vi "06.2 Handle Specific Errors Immediately.vi"() -> ()   [LabVIEW 2019]
uses:
  Support Files/02.4 DAQmx Configuration Cluster.ctl
  Support Files/03.2 States.ctl
  Support Files/03.2 State Machine Data.ctl
  <vilib>/DAQmx/read.llb/DAQmx Read (Analog 2D DBL NChan NSamp).vi
  <vilib>/DAQmx/write.llb/DAQmx Write (Analog DBL 1Chan 1Samp).vi
  <vilib>/DAQmx/create/channels.llb/DAQmx Create Channel (AI-Voltage-Basic).vi
  <vilib>/DAQmx/configure/timing.llb/DAQmx Timing (Sample Clock).vi
  <vilib>/DAQmx/miscellaneous.llb/DAQmx Fill In Error Info.vi
  <vilib>/Utility/file.llb/Write Delimited Spreadsheet (string).vi
  <vilib>/Utility/file.llb/Write Delimited Spreadsheet (DBL).vi
  <vilib>/DAQmx/create/channels.llb/DAQmx Create Channel (AO-Voltage-Basic).vi
panel:
  in  "DAQmx Configuration Cluster":T1={"Desired Sample Rate (Hz)"=-1.0, "sample mode"=10178, "Minimum value"=-1.0, "Maximum value"=-1.0, "Physical Channel"="", "units"=10143, "thermocouple type"=10072, "Samples per Channel"=0} {"thermocouple type" items=["J"=10072, "K"=10073, "N"=10077, "R"=10082, "S"=10085, "T"=10086, "B"=10047, "E"=10055]; "units" items=["Deg C"=10143, "Deg F"=10144, "Kelvins"=10325, "Deg R"=10145, "From Custom Scale"=10065]; "sample mode" items=["Finite Samples"=10178, "Continuous Samples"=10123, "Hardware Timed Single Point"=12522]}
  in  "Threshold (RMS)":dbl
  in  "Generate Stimulus":bool
  in  "Stop":bool
  in  "Clear":bool
  in  "Acquire":bool
  out "Graph":dbl[][](graph)
  out "Thershold Exceeded?":bool
  out "RMS Result per Channel":dbl[](array[numeric])
  # "ANALYSIS"
  # "EVENTS"
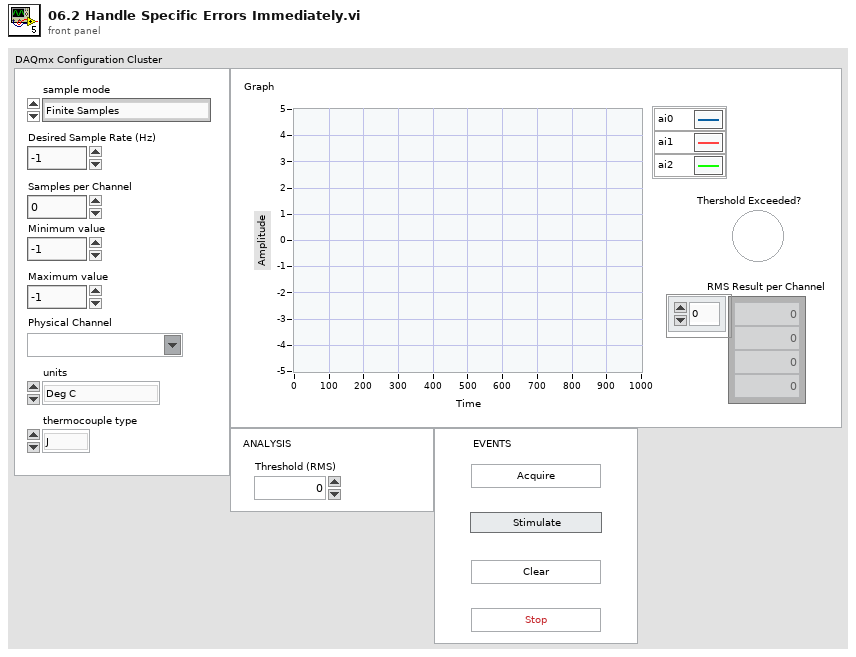
[diagram p1: front panel]
types:
  T1 = typedef "02.4 DAQmx Configuration Cluster.ctl" = cluster{"Desired Sample Rate (Hz)":dbl, "sample mode":i32, "Minimum value":dbl, "Maximum value":dbl, "Physical Channel":tag, "units":i32, "thermocouple type":i32, "Samples per Channel":i32}
  T2 = typedef "03.2 State Machine Data.ctl" = cluster{"Acquisition Data":dbl[][], "Stimulus?":bool}
  T3 = typedef "03.2 States.ctl" = enum16{"Initialize", "Update UI", "Update Stimulus", "Wait for event", "Acquire", "Analyze", "Log", "Clear", "Shutdown"}
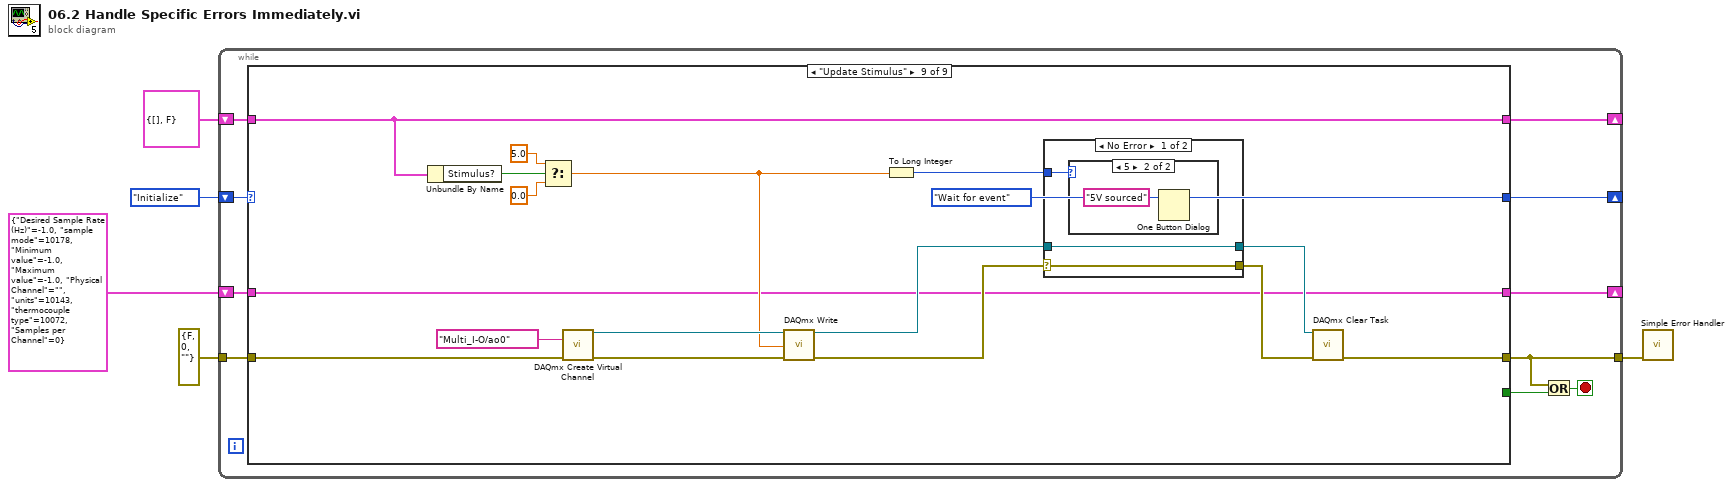
[diagram p0: block diagram]
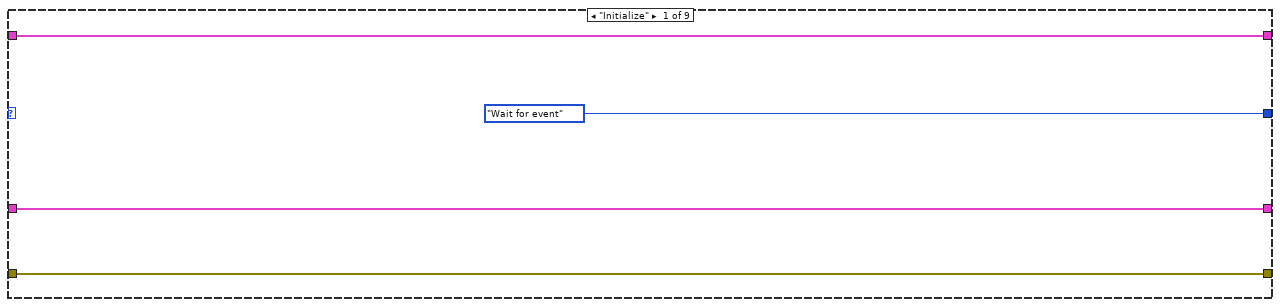
[diagram p2: hidden frame]
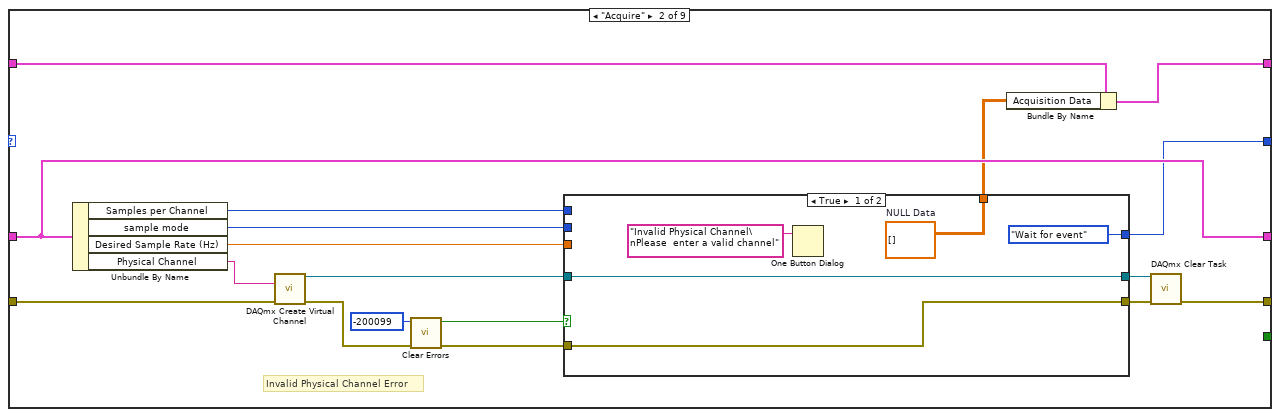
[diagram p3: hidden frame]
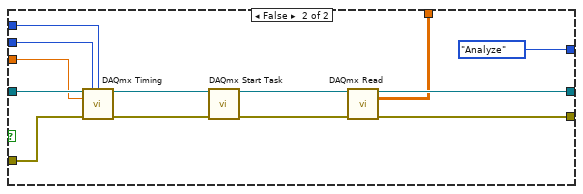
[diagram p4: hidden frame]
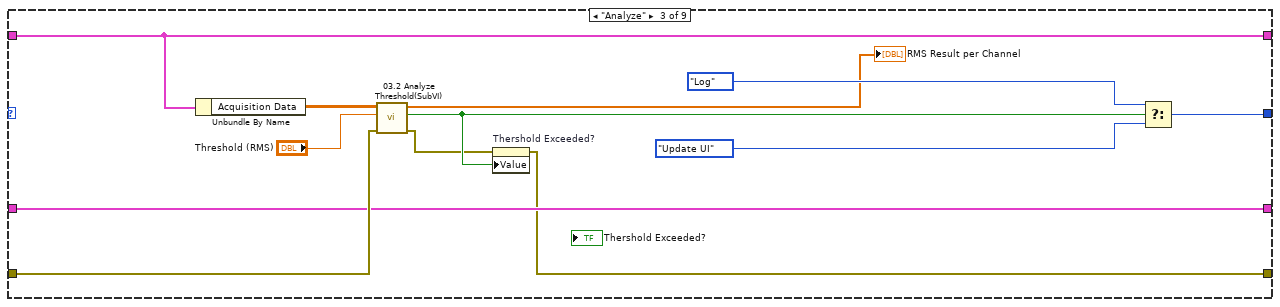
[diagram p5: hidden frame]
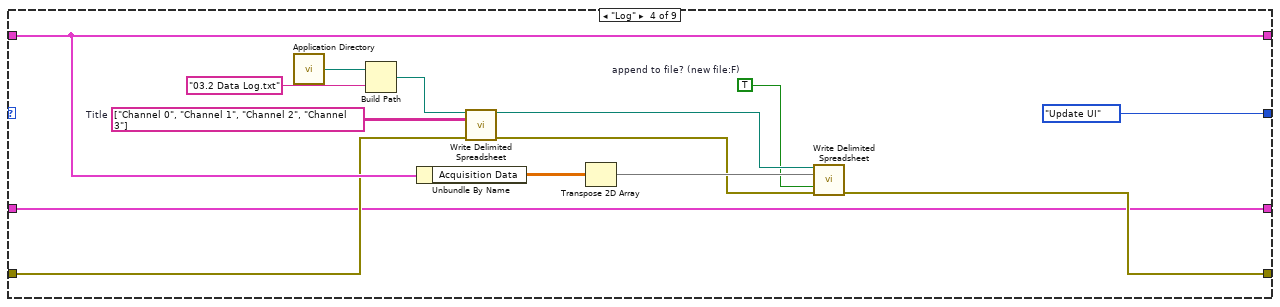
[diagram p6: hidden frame]
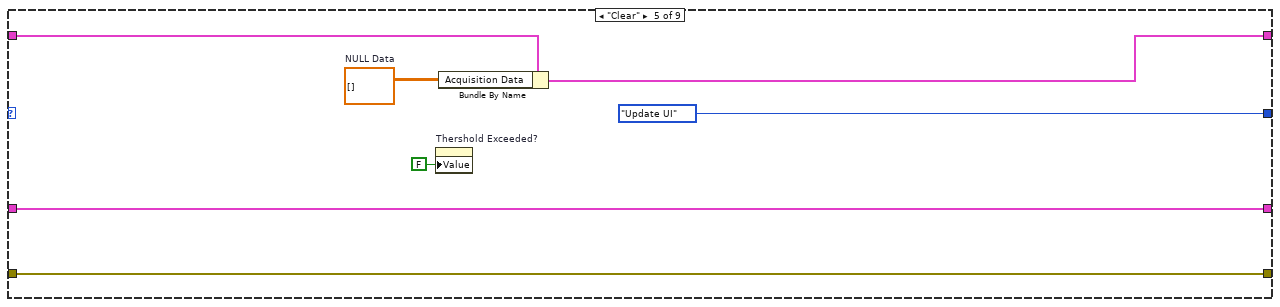
[diagram p7: hidden frame]
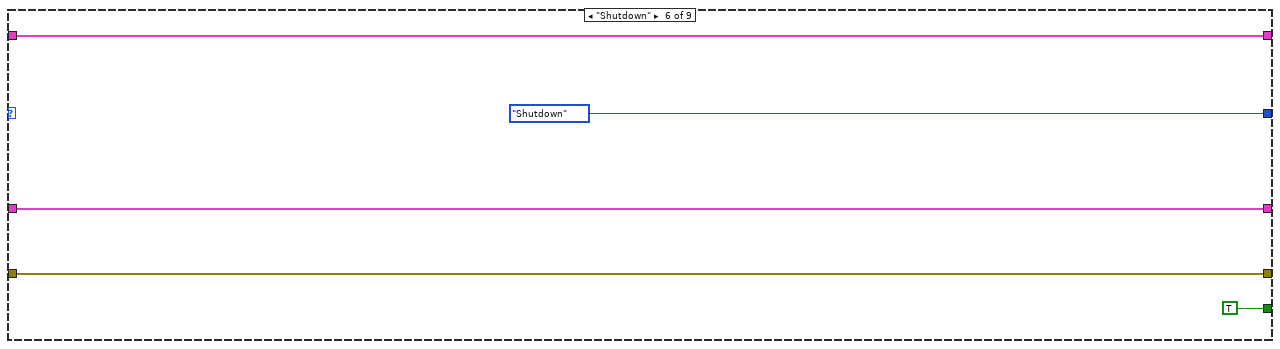
[diagram p8: hidden frame]
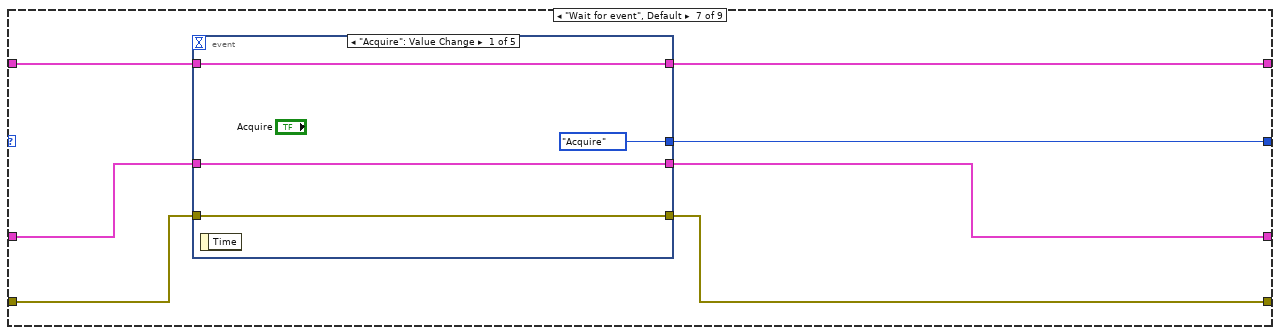
[diagram p9: hidden frame]
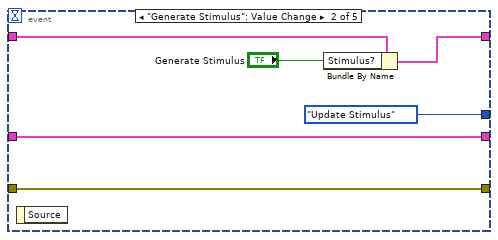
[diagram p10: hidden frame]
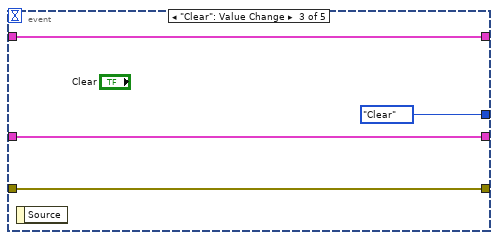
[diagram p11: hidden frame]
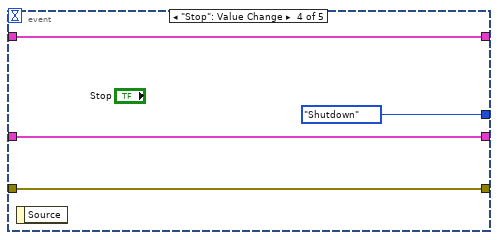
[diagram p12: hidden frame]
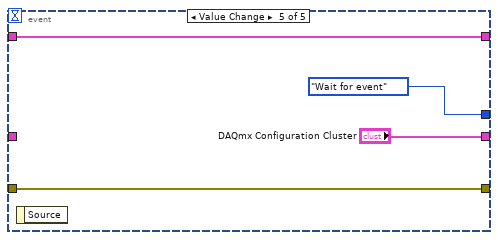
[diagram p13: hidden frame]
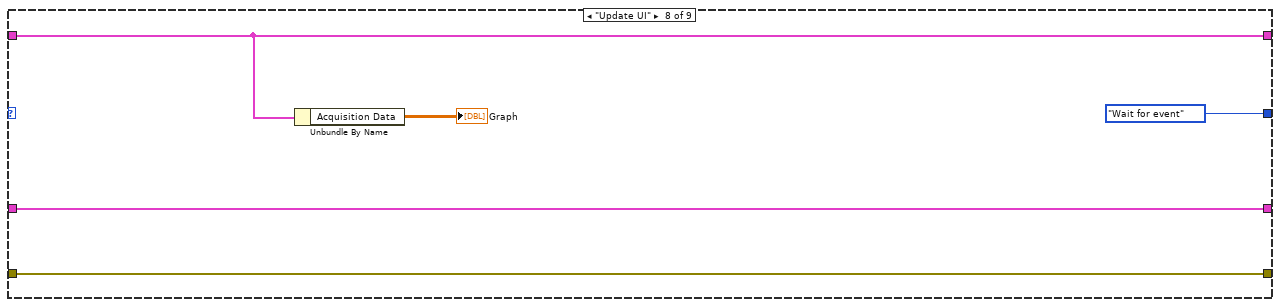
[diagram p14: hidden frame]
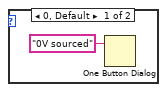
[diagram p15: hidden frame]
diagram:
  n1 = while {
    shift-right: [w14] -> _
    shift-left: 03.2_States."Initialize" ("State") -> [w15]
    tunnel: errorcluster {"status"=FALSE, "code"=0, "source"=""} ("error constant") -> [w13]
    tunnel: [w11] -> w3
    shift-right: [w10] -> _
    shift-left: T2 {"Acquisition Data"=[], "Stimulus?"=FALSE} -> [w9]
    shift-right: [w6] -> _
    shift-left: T1 {"Desired Sample Rate (Hz)"=-1.0, "sample mode"=10178, "Minimum value"=-1.0, "Maximum value"=-1.0, "Physical Channel"="", "units"=10143, "thermocouple type"=10072, "Samples per Channel"=0} ("DAQmx Configuration Cluster") -> [w7]
    stop <- w12 stop-if-true
    n2 = case shown="\"Update Stimulus\"" w15 {
      tunnel: [03.2_States."Wait for event" ("State") w20 w66 03.2_States."Update UI" ("State") 03.2_States."Update UI" ("State") 03.2_States."Shutdown" ("State") w100 03.2_States."Wait for event" ("State") 03.2_States."Wait for event" ("State")] -> w14
      tunnel: [w18 w27 w56 w79 w84 w91 w99 w125 w133] -> w11
      tunnel: w13 -> [w18 w32 w63 w69 w84 w91 w98 w125 w144]
      tunnel: [w19 w21 w62 w77 w87 w92 w97 w127 w130] -> w10
      tunnel: w9 -> [w19 w23 w62 w77 w88 w92 w96 w127 w130]
      tunnel: [_ _ _ _ _ TRUE _ _ _] -> w8
      tunnel: w7 -> [w16 w24 w58 w68 w83 w89 w95 w123 w129]
      tunnel: [w16 w24 w58 w68 w83 w89 w94 w123 w129] -> w6
      frame "Initialize" {
      }
      frame "Acquire" {
        # "Invalid Physical Channel Error"
        n3 = Unbundle By Name(w24) -> ("Samples per Channel"=w34:i32, "sample mode"=w35:i32, "Desired Sample Rate (Hz)"=w36:dbl, "Physical Channel"=w33:tag)
        n4 = call-poly <vilib>:"DAQmx Create Virtual Channel.vi"("physical channels"=w33, "error in"=w32) -> ("task out"=w37:refnum<k21>, "error out"=w31:errorcluster)  [unwired: 12 in]
        n5 = call <vilib>:"Clear Errors.vi"("error in (no error)"=w31, "specific error code to clear (0: all)"=-200099) -> ("error out"=w29:errorcluster, "specific error cleared?"=w28:bool)  [unwired: 4 in]
        n6 = case shown="True" w28 {
          tunnel: w29 -> [w41 w55]
          tunnel: w37 -> [w42 w54]
          tunnel: w36 -> [_ w49]
          tunnel: w35 -> [_ w48]
          tunnel: w34 -> [_ w47]
          tunnel: [w41 w46] -> w26
          tunnel: [w42 w45] -> w25
          tunnel: [w40 w44] -> w22
          tunnel: [03.2_States."Wait for event" ("State") 03.2_States."Analyze" ("State")] -> w20
          frame True {
            w40 = dbl[][] []  # NULL Data
            n7 = One Button Dialog(message="Invalid Physical Channel\nPlease  enter a valid channel") -> ()  [unwired: 1 in, 1 out]
          }
          frame False {
            n8 = call-poly <vilib>:"DAQmx Timing.vi"("task/channels in"=w54, "sample mode"=w48, "samples per channel"=w47, "rate"=w49, "error in"=w55) -> ("task out"=w50:refnum<k21>, "error out"=w51:errorcluster)  [unwired: 9 in]
            n9 = call <vilib>:"DAQmx Start Task.vi"("task/channels in"=w50, "error in"=w51) -> ("task out"=w52:refnum<k21>, "error out"=w53:errorcluster)  [unwired: 12 in]
            n10 = call-poly <vilib>:"DAQmx Read.vi"("task/channels in"=w52, "error in"=w53) -> ("task out"=w45:refnum<k21>, "data"=w44:dbl[][], "error out"=w46:errorcluster)  [unwired: 11 in]
          }
        }
        n11 = Bundle By Name(cluster=w23, "Acquisition Data"=w22) -> (w21:T2)
        n12 = call <vilib>:"DAQmx Clear Task.vi"("task in"=w25, "error in"=w26) -> ("error out"=w27:errorcluster)  [unwired: 13 in]
      }
      frame "Analyze" {
        n13 = Unbundle By Name(w62) -> ("Acquisition Data"=w67:dbl[][])
        n14 = call "03.2 Analyze Threshold(SubVI).vi"("Error In"=w63, "Threshold (RMS)"="Threshold (RMS)", "Data"=w67) -> ("Error Out"=w57:errorcluster, "Threshold exceeded?"=w59:bool, "RMS Results per Channel"=→"RMS Result per Channel":dbl[])  [unwired: 6 in]
        n15 = property on="Thershold Exceeded?" class="Bool (strict)"(error in=w57, "Value"=w59) -> (error out=w56:errorcluster)  [unwired: 1 in, 1 out]
        n16 = Select(t=03.2_States."Log" ("State"), s=w59, f=03.2_States."Update UI" ("State")) -> (s? t:f=w66:T3)
      }
      frame "Log" {
        w71 = string[][] [["Channel 0", "Channel 1", "Channel 2", "Channel 3"]]  # Title
        w73 = TRUE  # append to file? (new file:F)
        n17 = call <vilib>:"Application Directory.vi"() -> ("Application Directory"=w81:path)
        n18 = Build Path(base path=w81, name or relative path="03.2 Data Log.txt") -> (appended path=w72:path)
        n19 = Unbundle By Name(w77) -> ("Acquisition Data"=w76:dbl[][])
        n20 = call-poly <vilib>:"Write Delimited Spreadsheet.vi"("file path (dialog if empty)"=w72, "2D data"=w71, "error in (no error)"=w69) -> ("new file path (Not A Path if cancelled)"=w74:path, "error out"=w70:errorcluster)  [unwired: 11 in]
        n21 = Transpose 2D Array(2D array=w76) -> (transposed array=w75:dbl[][])
        n22 = call-poly <vilib>:"Write Delimited Spreadsheet.vi"("file path (dialog if empty)"=w74, "2D data"=w75, "append to file? (new file:F)"=w73, "error in (no error)"=w70) -> ("error out"=w79:errorcluster)  [unwired: 10 in, 1 out]
      }
      frame "Clear" {
        w86 = dbl[][] []  # NULL Data
        n23 = property on="Thershold Exceeded?" class="Bool (strict)"("Value"=FALSE ("Thershold Exceeded?")) -> ()  [unwired: 2 in, 2 out]
        n24 = Bundle By Name(cluster=w88, "Acquisition Data"=w86) -> (w87:T2)
      }
      frame "Shutdown" {
      }
      frame "Wait for event", Default {
        n25 = event shown="[0] \"Acquire\": Value Change" {
          selector: _ -> [_ _ _ _ _]
          dyn-events: _ -> [_ _ _ _ _]
          timeout: _ -> [_ _ _ _ _]
          tunnel: [03.2_States."Acquire" ("State") 03.2_States."Update Stimulus" ("State") 03.2_States."Clear" ("State") 03.2_States."Shutdown" ("State") 03.2_States."Wait for event" ("State")] -> w100
          tunnel: [w103 w106 w112 w117 w119] -> w99
          tunnel: w98 -> [w103 w106 w112 w117 w119]
          tunnel: [w102 w108 w114 w116 w121] -> w97
          tunnel: w96 -> [w102 w110 w114 w116 w121]
          tunnel: w95 -> [w101 w105 w111 w115 _]
          tunnel: [w101 w105 w111 w115 "DAQmx Configuration Cluster"] -> w94
          event "Acquire": Value Change {
            n26 = event-data() -> ()  [unwired: 1 in, 1 out]
          }
          event "Generate Stimulus": Value Change {
            n27 = event-data() -> ()  [unwired: 1 in, 1 out]
            n28 = Bundle By Name(cluster=w110, "Stimulus?"="Generate Stimulus") -> (w108:T2)
          }
          event "Clear": Value Change {
            n29 = event-data() -> ()  [unwired: 1 in, 1 out]
          }
          event "Stop": Value Change {
            n30 = event-data() -> ()  [unwired: 1 in, 1 out]
          }
          event Value Change {
            n31 = event-data() -> ()  [unwired: 1 in, 1 out]
          }
        }
      }
      frame "Update UI" {
        n32 = Unbundle By Name(w127) -> ("Acquisition Data"=→"Graph":dbl[][])
      }
      frame "Update Stimulus" {
        n33 = Unbundle By Name(w130) -> ("Stimulus?"=w141:bool)
        n34 = Select(t=5.0, s=w141, f=0.0) -> (s? t:f=w138:dbl)
        n35 = call-poly <vilib>:"DAQmx Create Virtual Channel.vi"("physical channels"=tag "Multi_I-O/ao0", "error in"=w144) -> ("task out"=w142:refnum<k21>, "error out"=w143:errorcluster)  [unwired: 12 in]
        n36 = call-poly <vilib>:"DAQmx Write.vi"("task/channels in"=w142, "data"=w138, "error in"=w143) -> ("task out"=w136:refnum<k21>, "error out"=w137:errorcluster)  [unwired: 10 in, 1 out]
        n37 = To Long Integer(number=w138) -> (32bit integer=w131:i32)
        n38 = case shown="No Error" w137 {
          selector: w137 -> [w147 w150]
          tunnel: w136 -> [w146 w151]
          tunnel: [w147 w150] -> w135
          tunnel: [w146 w151] -> w134
          tunnel: w131 -> [w145 _]
          frame No Error {
            n39 = case shown="5" w145 {
              frame 0, Default {
                n40 = One Button Dialog(message="0V sourced") -> ()  [unwired: 1 in, 1 out]
              }
              frame 5 {
                n41 = One Button Dialog(message="5V sourced") -> ()  [unwired: 1 in, 1 out]
              }
            }
          }
          frame Error {
          }
        }
        n42 = call <vilib>:"DAQmx Clear Task.vi"("task in"=w134, "error in"=w135) -> ("error out"=w133:errorcluster)  [unwired: 13 in]
      }
    }
    n43 = Or(x=w11, y=w8) -> (x .or. y?=w12:bool)
  }
  n44 = call <vilib>:"Simple Error Handler.vi"("error in (no error)"=w3) -> ()  [unwired: 4 in, 5 out]
